vi "myRIO_BRig_RT__Case_Exp_State_Selection__v2.vi"(0 "input_dataCurrent":u16[](array[numeric]), 1 "input_state":T1, 7 "input_FPGA_SelectReward":bool, 9 "input_FPGA_SelectWrong":bool, 12 "input_arrTrig":bool[](array[boolean])) -> (3 "output_state":T1, 4 "output_dataCurrent":u16[](array[numeric]), 10 "output_LC_Event_l1":bool, 13 "output_LC_Laser_l2":bool, 14 "output_LC_Event_l2":bool, 15 "output_LC_Laser_l1":bool)   [LabVIEW 2014]
uses:
  myRIO_BRig_RT__Case_Exp_stateList.ctl
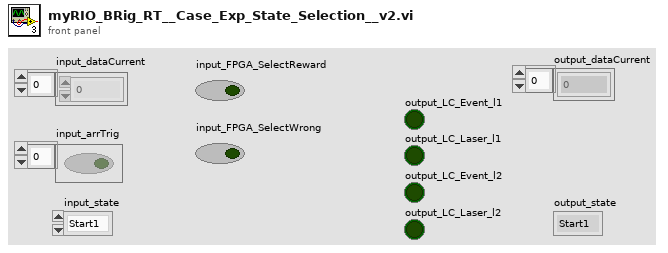
[diagram p1: front panel]
types:
  T1 = typedef "myRIO_BRig_RT__Case_Exp_stateList.ctl" = enum16{"Start1", "Start2", "Start3", "saveSettings1", "saveSettings2", "saveSettings3", "saveSettings4", "saveSettings_LC_ENL_l1", "saveSettings_LC_ENL_l2", "saveSettings_LC_Cue_l1", "saveSettings_LC_Cue_l2", "saveSettings6_LC_l1_Other", "SaveSettings6_LC_l2_Other", "setSettings_Audio", "setSettings_Laser", "initBlock_pre", "initBlock", "initBlock2", "initBlock_post", "initTrial_pre", "initTrial", "initTrial2", "initTrial3", "initTrial4", "initTrial_LC_ENL1", "initTrial_LC_Cue1", "initTrial_LC_Cue1_2", "initTrial_LC_Sel", "initTrial_post", "ENL1_pre", "ENL1", "ENL1_post", "ENL1Penalty_pre", "ENL1Penalty", "ENL2_pre", "ENL2", "ENL2Penalty_pre", "ENL2Penalty", "Cue1_pre", "Cue1", "Cue1_post", "Cue1Penalty_pre", "Cue1Penalty", "Cue2_pre", "Cue2", "Cue2Penalty_pre", "Cue2Penalty", "Selection_pre", "Selection", "Select_post", "SelectReward_pre", "SelectReward", "SelectRewardPost_pre", "SelectRewardPost", "SelectWrong_pre", "SelectWrong", "SelectWrong_post", "SelectTimeout_pre", "SelectTimeout", "SelectTimeout_post", "endTrial_pre", "endTrial1", "endTrial2", "endTrial3", "endTrial_post", "endBlock_pre", "endBlock", "endBlock_post", "endExp", "commConnect", "commUpload_pre", "commUpload_dataBlock", "commUpload_dataCurrent", "commUpload_dataExp", "commUpload_dataLC", "commUpload_dataTrial", "commUpload_post", "saveData_pre", "saveData_dataBlock", "saveData_dataCurrent", "saveData_dataExp", "saveData_dataLC", "saveData_dataTrial", "saveData_post", "empty_endBlock1", "empty_endBlock2", "empty_endTrial1", "empty_endTrial2", "empty_endTrial3", "empty_endTrial4", "empty_endTrial5", "dummyState", "dummyState_endBlock"}
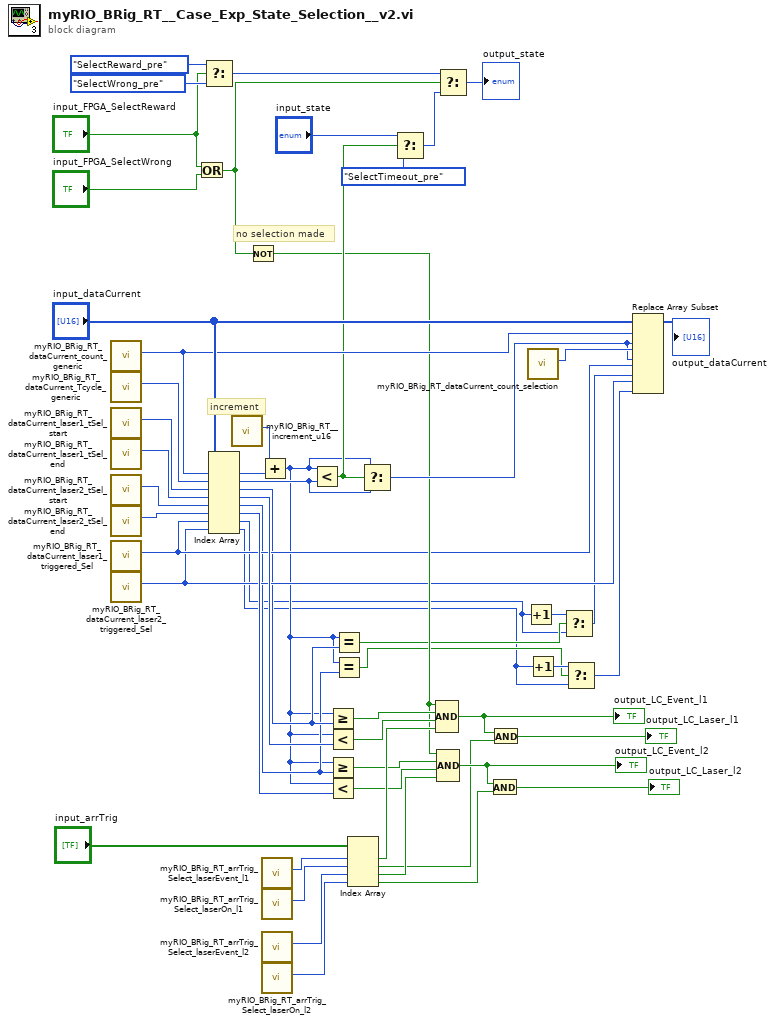
[diagram p0: block diagram]
diagram:
  # "no selection made"
  # "increment"
  n1 = call "myRIO_BRig_RT_dataCurrent_count_generic.vi"() -> ("output_count_generic"=w38:i32)  [unwired: 11 in]
  n2 = call "myRIO_BRig_RT_dataCurrent_Tcycle_generic.vi"() -> ("output_Tcycle_generic"=w50:i32)  [unwired: 11 in]
  n3 = call "myRIO_BRig_RT_dataCurrent_laser1_tSel_start.vi"() -> ("output_laser1_tSel_start"=w51:i32)  [unwired: 11 in]
  n4 = call "myRIO_BRig_RT_dataCurrent_laser1_tSel_end.vi"() -> ("output_laser1_tSel_end"=w52:i32)  [unwired: 11 in]
  n5 = call "myRIO_BRig_RT_dataCurrent_laser2_tSel_start.vi"() -> ("output_laser2_tSel_start"=w43:i32)  [unwired: 11 in]
  n6 = call "myRIO_BRig_RT_dataCurrent_laser2_tSel_end.vi"() -> ("output_laser2_tSel_end"=w42:i32)  [unwired: 11 in]
  n7 = call "myRIO_BRig_RT_dataCurrent_laser1_triggered_Sel.vi"() -> ("output_laser1_triggered_Selection"=w13:i32)  [unwired: 11 in]
  n8 = call "myRIO_BRig_RT_dataCurrent_laser2_triggered_Sel.vi"() -> ("output_laser2_triggered_Selection"=w12:i32)  [unwired: 11 in]
  n9 = Or(x="input_FPGA_SelectReward", y="input_FPGA_SelectWrong") -> (x .or. y?=w32:bool)
  n10 = Select(t=myRIO_BRig_RT__Case_Exp_stateList."SelectReward_pre" ("Enum"), s="input_FPGA_SelectReward", f=myRIO_BRig_RT__Case_Exp_stateList."SelectWrong_pre" ("Enum")) -> (s? t:f=w53:T1)
  n11 = Index Array(array="input_dataCurrent", index #1=w38, index #2=w50, index #3=w51, index #4=w52, index #5=w43, index #6=w42, index #7=w13, index #8=w12) -> (element #1=w48:u16, element #2=w36:u16, element #3=w11:u16, element #4=w41:u16, element #5=w10:u16, element #6=w40:u16, element #7=w6:u16, element #8=w3:u16)
  n12 = call "myRIO_BRig_RT__increment_u16.vi"() -> ("output_increment__u16"=w49:u16)  [unwired: 11 in]
  n13 = Not(x=w32) -> (.not. x?=w25:bool)
  n14 = Add(x=w49, y=w48) -> (x+y=w9:u16)
  n15 = call "myRIO_BRig_RT_arrTrig_Select_laserEvent_l1.vi"() -> ("output_arrTrig_Select_laserEvent_l1"=w28:i32)  [unwired: 11 in]
  n16 = call "myRIO_BRig_RT_arrTrig_Select_laserOn_l1.vi"() -> ("output_arrTrig_Select_laserOn_l1"=w27:i32)  [unwired: 11 in]
  n17 = call "myRIO_BRig_RT_arrTrig_Select_laserEvent_l2.vi"() -> ("output_arrTrig_Select_laserEvent_l2"=w15:i32)  [unwired: 11 in]
  n18 = call "myRIO_BRig_RT_arrTrig_Select_laserOn_l2.vi"() -> ("output_arrTrig_Select_laserOn_l2"=w14:i32)  [unwired: 11 in]
  n19 = Less?(x=w9, y=w36) -> (x < y?=w37:bool)
  n20 = Greater Or Equal?(x=w9, y=w11) -> (x >= y?=w31:bool)
  n21 = Less?(x=w9, y=w41) -> (x < y?=w30:bool)
  n22 = Greater Or Equal?(x=w9, y=w10) -> (x >= y?=w24:bool)
  n23 = Less?(x=w9, y=w40) -> (x < y?=w23:bool)
  n24 = Equal?(x=w9, y=w11) -> (x = y?=w8:bool)
  n25 = Equal?(x=w9, y=w10) -> (x = y?=w4:bool)
  n26 = Index Array(array="input_arrTrig", index #1=w28, index #2=w27, index #3=w15, index #4=w14) -> (element #1=w26:bool, element #2=w18:bool, element #3=w22:bool, element #4=w20:bool)
  n27 = Select(t=w9, s=w37, f=w36) -> (s? t:f=w34:u16)
  n28 = Select(t="input_state", s=w37, f=myRIO_BRig_RT__Case_Exp_stateList."SelectTimeout_pre" ("Enum")) -> (s? t:f=w45:T1)
  n29 = Compound Arithmetic op=AND(w25, w31, w30, w26) -> (w19:bool)
  "output_LC_Event_l1" <- w19
  n30 = Compound Arithmetic op=AND(w25, w24, w23, w22) -> (w21:bool)
  "output_LC_Event_l2" <- w21
  n31 = Select(t=w53, s=w32, f=w45) -> (s? t:f=→"output_state":T1)
  n32 = And(x=w21, y=w20) -> (x .and. y?=→"output_LC_Laser_l2":bool)
  n33 = And(x=w19, y=w18) -> (x .and. y?=→"output_LC_Laser_l1":bool)
  n34 = Increment(x=w6) -> (x+1=w7:u16)
  n35 = call "myRIO_BRig_RT_dataCurrent_count_selection.vi"() -> ("output_count_generic"=w35:i32)  [unwired: 11 in]
  n36 = Increment(x=w3) -> (x+1=w5:u16)
  n37 = Select(t=w7, s=w8, f=w6) -> (s? t:f=w2:u16)
  n38 = Select(t=w5, s=w4, f=w3) -> (s? t:f=w1:u16)
  n39 = Replace Array Subset(array="input_dataCurrent", new element #1=w34, index #1=w38, new element #2=w34, index #2=w35, new element #3=w2, index #3=w13, new element #4=w1, index #4=w12) -> (→"output_dataCurrent":u16[])
